vi "HapticSTM_FBL.vi"() -> ()   [LabVIEW 2019]
uses:
  <userlib>/HapticSTM/HapticSTM.lvlib
  SubVIs/GlobalClicksHeight_FBL.vi
  <vilib>/sound2/lvsound2.llb/Sampling Mode.ctl
  <vilib>/sound2/lvsound2.llb/Sound Data Format.ctl
  <vilib>/sound2/lvsound2.llb/Sound Output Write (DBL Single).vi
  <vilib>/sound2/lvsound2.llb/Sound Output Set Volume (Single).vi
panel:
  in  "Surface Location (nm)":dbl
  in  "Z Write?":bool
  in  "Planing?":bool
  in  "Plunge Depth (pm)":dbl=280.0 format="%.1f"
  out "Button":bool
  out "Setpoint (pA)":dbl
  in  "Maximum (pA)":dbl=9000.0
  out "Filtered Current (pA)":dbl format="%.1f"
  out "Current (pA)":dbl format="%.1f"
  out "Oy":dbl
  out "Ox":dbl
  out "W":dbl
  out "H":dbl
  out "Z Write (m)":dbl format="%^.1e"
  out "Z Read (m)":dbl format="%^#.1e"
  out "Vy":dbl format="%.1f"
  out "Vz":dbl format="%.1f"
  out "Vx":dbl format="%.1f"
  out "Fy":dbl format="%.1f"
  out "Fz":dbl format="%.1f"
  out "Fx":dbl format="%.1f"
  out "phi":dbl format="%.1f"
  out "psi":dbl format="%.1f"
  out "theta":dbl format="%.1f"
  out "x":dbl format="%.1f"
  out "y":dbl format="%.1f"
  out "z":dbl format="%0.1f"
  out "Height":dbl format="%^.1e"
  in  "Hardness":dbl=1.0 format="%.1f"
  in  "Mode":u16(ring) items=["Log w/ Exp Z", "Log w/ Lin Z"]
  in  "Reset Clicks":bool
  out "Clicks":i32
  in  "STOP":bool
  in  "START":bool
  out "Seq":i32
  out "SeqString":string
  out "Raw and Scaled Z Positions":cluster{dbl, "Y":dbl}(graph)
  out "Scaled Force and Current":T1(graph)
  in  "Sensitivity":dbl=1.0 format="%.1f"
  in  "Volume":dbl(slide)=50.0 scale=0.0..100.0
  in  "Device ID":u32
  # "Nanonis"
  # "No"
  # "Yes"
  # "Current"
  # "Frame"
  # "Z Controller"
  # "Haptic Pen"
  # "Position"
  # "Force"
  # "Angles"
  # "Velocity"
  # "Surface"
  # "Clicks"
  # "Haptic STM Controller 3000"
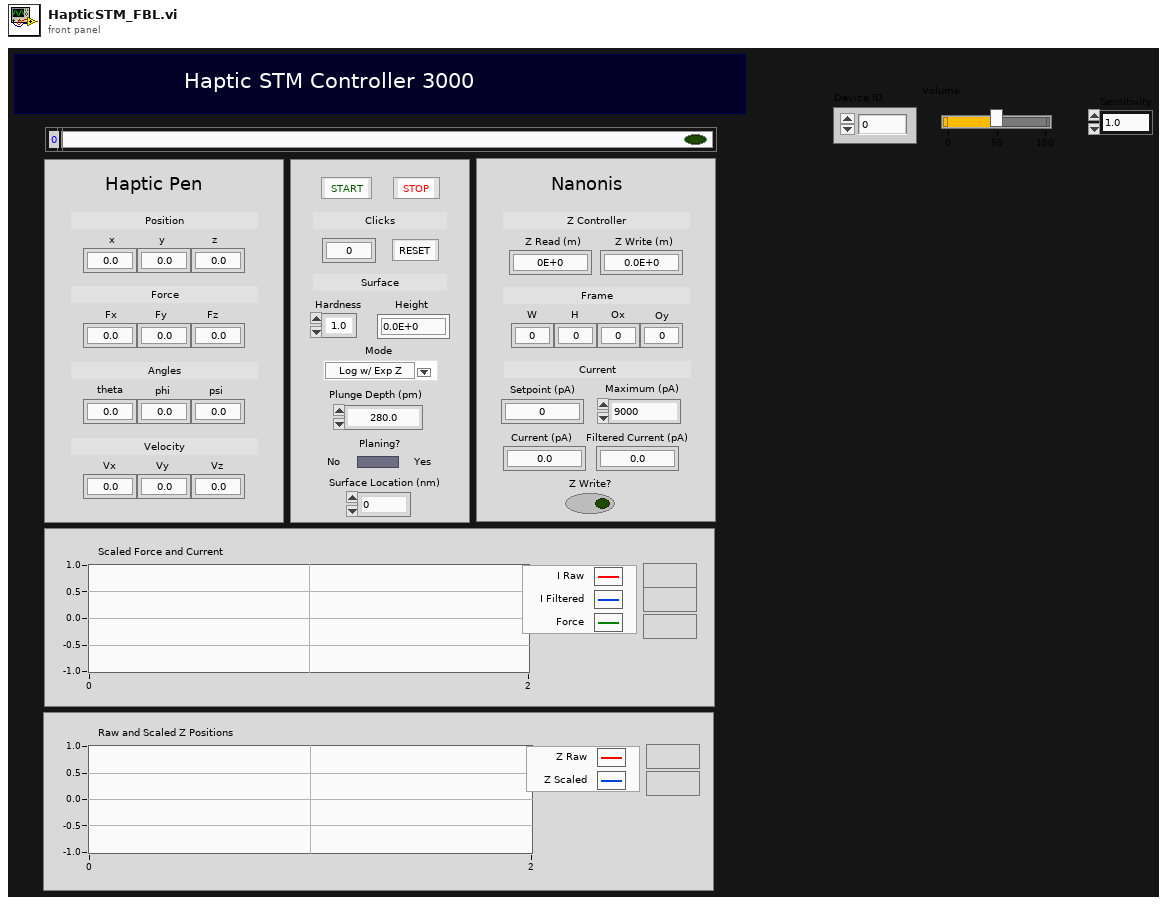
[diagram p1: front panel]
types:
  T1 = cluster{"Current (pA)":sgl, "Filtered Current (pA)":dbl, dbl}
  T2 = typedef "Sound Data Format.ctl" = cluster{"sample rate (S/s)":dbl, "number of channels":i32, "bits per sample":i32}
  T3 = typedef "Sampling Mode.ctl" = i32
  T4 = typedef "Sound Output Task ID.ctl" = u32
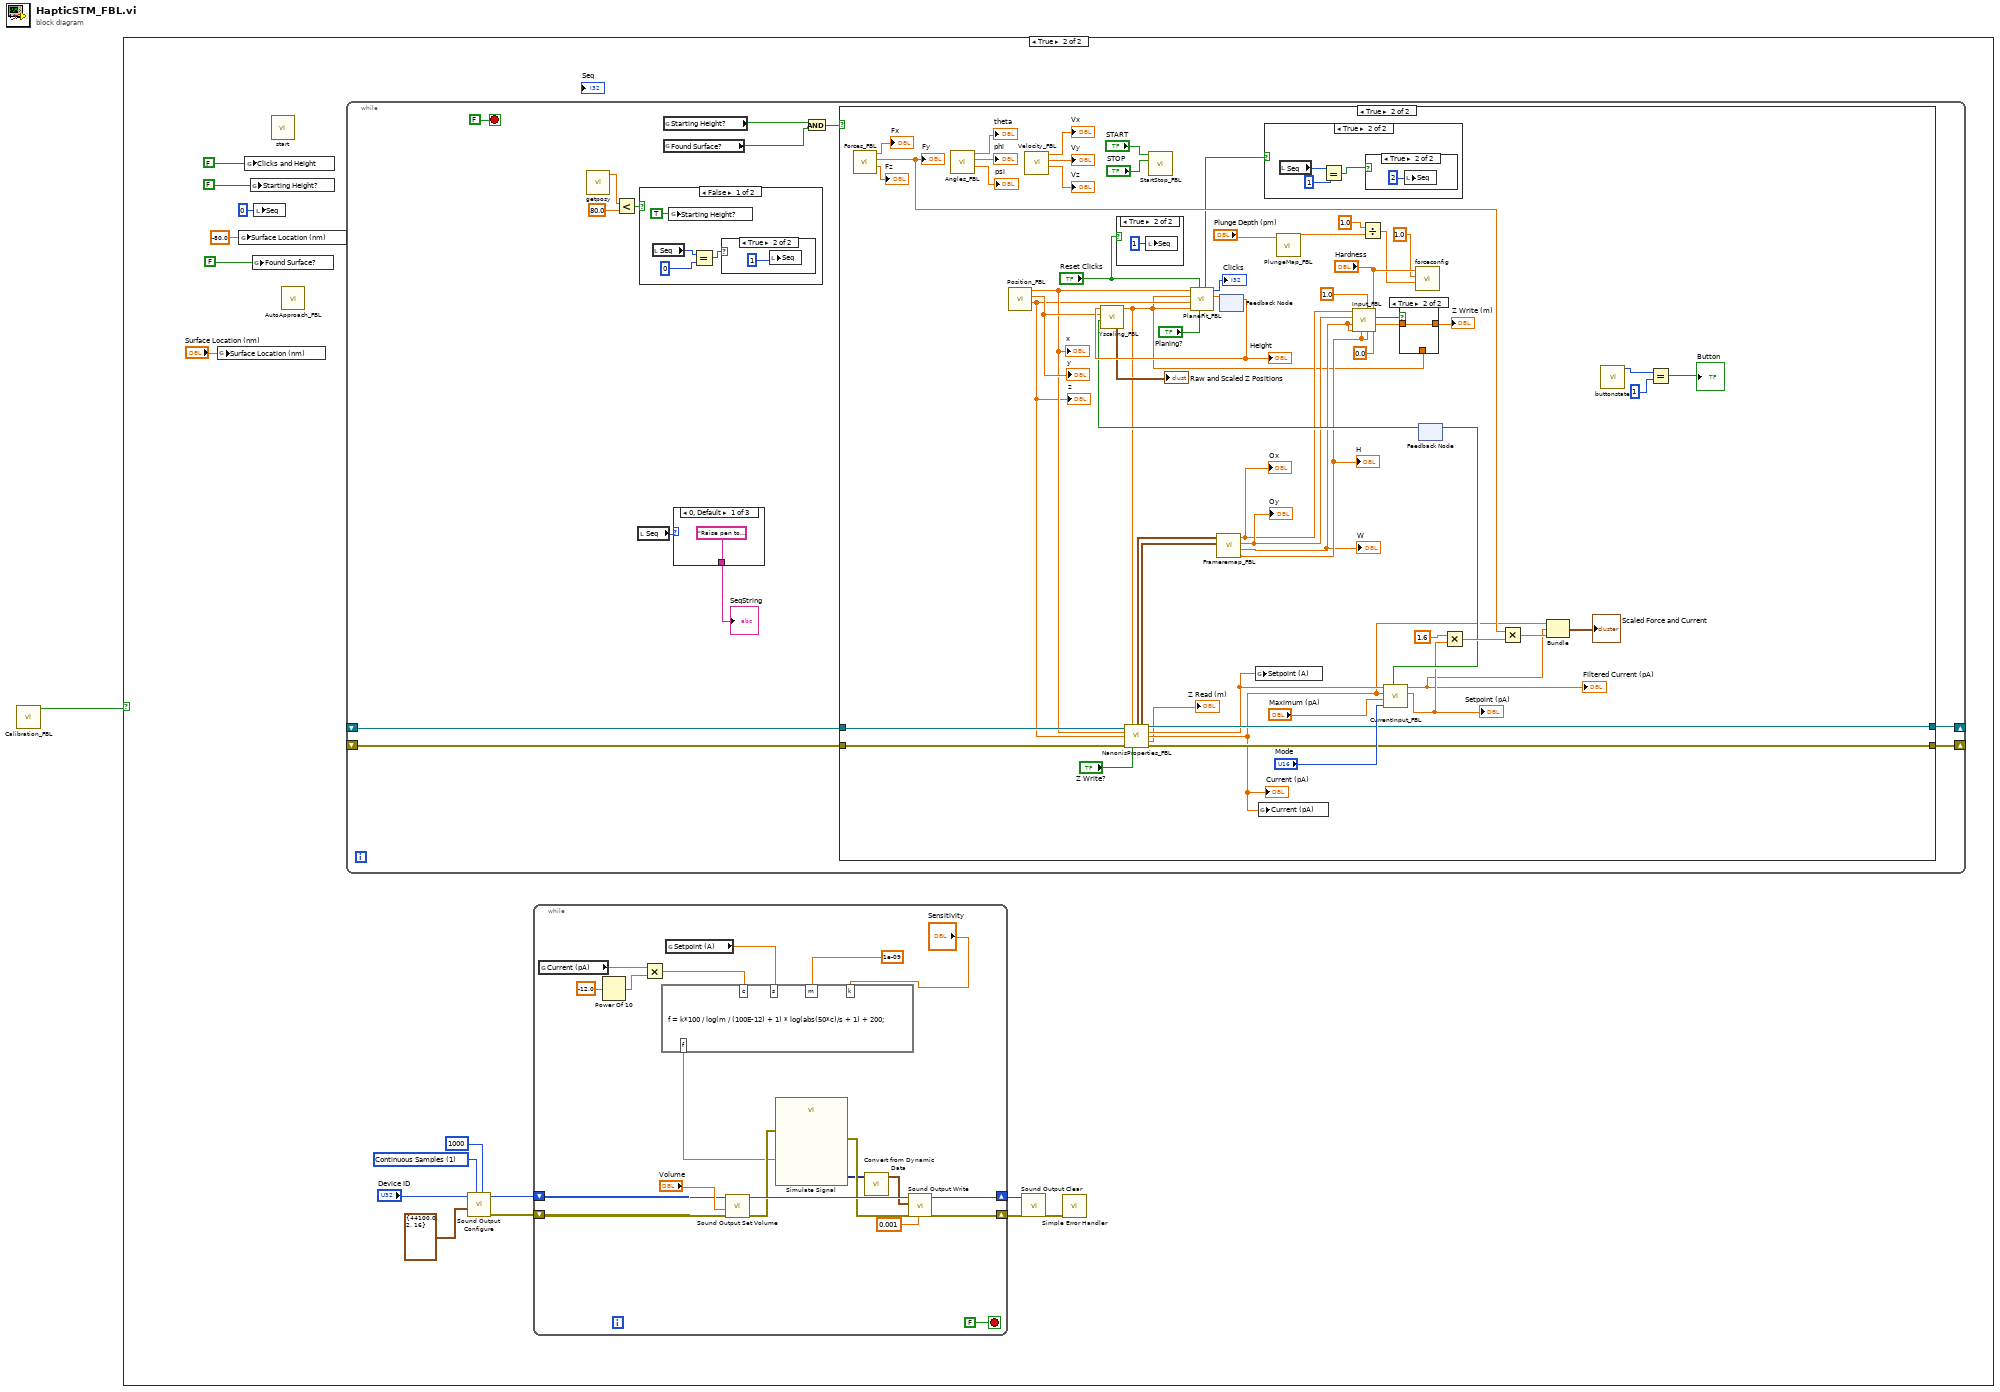
[diagram p0: block diagram]
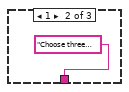
[diagram p3: hidden frame]
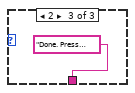
[diagram p4: hidden frame]
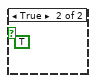
[diagram p6: hidden frame]
diagram:
  n1 = call "Calibration_FBL.vi"() -> ("Calibration Complete?"=w1:bool)  [unwired: 11 in]
  n2 = case shown="True" w1 {
    frame False {
    }
    frame True {
      w10 = T3 1 items=["Finite Samples", "Continuous Samples"] ("sample mode")
      n3 = global write "GlobalClicksHeight_FBL.vi" "Surface Location (nm)"("Surface Location (nm)") -> ()
      n4 = global write "GlobalClicksHeight_FBL.vi" "Surface Location (nm)"(-80.0 ("Surface Location")) -> ()
      n5 = global write "GlobalClicksHeight_FBL.vi" "Clicks and Height"(FALSE ("Clicks and Height")) -> ()
      n6 = global write "GlobalClicksHeight_FBL.vi" "Starting Height?"(FALSE ("Clicks and Height")) -> ()
      n7 = global write "GlobalClicksHeight_FBL.vi" "Found Surface?"(FALSE ("Clicks and Height")) -> ()
      n8 = local write "Seq"(0 ("Seq")) -> ()
      n9 = call <userlib>:"start.vi"() -> ()  [unwired: 11 in, 1 out]
      n10 = call "AutoApproach_FBL.vi"() -> ()  [unwired: 12 in]
      n11 = while {
        shift-right: [w39] -> _
        shift-left: _ -> [w40]
        shift-right: [w38] -> _
        shift-left: _ -> [w37]
        stop <- FALSE stop-if-true
        n12 = call <userlib>:"getposy.vi"() -> ("function return"=w49:dbl)  [unwired: 11 in]
        n13 = Less?(x=w49, y=80.0) -> (x < y?=w47:bool)
        n14 = local read "Seq"() -> (w45:i32)
        n15 = case shown="False" w47 {
          frame False {
            n16 = local read "Seq"() -> (w55:i32)
            n17 = global write "GlobalClicksHeight_FBL.vi" "Starting Height?"(TRUE ("Starting Height?")) -> ()
            n18 = Equal?(x=w55, y=0) -> (x = y?=w53:bool)
            n19 = case shown="True" w53 {
              frame False {
              }
              frame True {
                n20 = local write "Seq"(1 ("Seq")) -> ()
              }
            }
          }
          frame True {
            (unwired) TRUE ("Clicks and Height")
          }
        }
        n21 = global read "GlobalClicksHeight_FBL.vi" "Starting Height?"() -> (w42:bool)
        n22 = global read "GlobalClicksHeight_FBL.vi" "Found Surface?"() -> (w41:bool)
        n23 = case shown="0, Default" w45 {
          tunnel: ["Raise pen to begin." "Choose three points, then raise the arm to plane." "Done. Press 'STOP' to stop at anytime."] -> w44
          frame 0, Default {
          }
          frame 1 {
          }
          frame 2 {
          }
        }
        "SeqString" <- w44
        n24 = And(x=w42, y=w41) -> (x .and. y?=w43:bool)
        n25 = case shown="True" w43 {
          tunnel: w40 -> [_ w72]
          tunnel: [_ w71] -> w39
          tunnel: [_ w70] -> w38
          tunnel: w37 -> [_ w69]
          frame False {
          }
          frame True {
            n26 = call "Forces_FBL.vi"() -> ("Fz"=→"Fz":dbl, "Fy"=w102:dbl, "Fx"=→"Fx":dbl)  [unwired: 9 in]
            "Fy" <- w102
            n27 = call "Angles_FBL.vi"() -> ("psi"=→"psi":dbl, "phi"=→"phi":dbl, "theta"=→"theta":dbl)  [unwired: 9 in]
            n28 = call "Position_FBL.vi"() -> ("Z"=w67:dbl, "Y"=w98:dbl, "X"=w68:dbl)  [unwired: 9 in]
            "x" <- w68
            "y" <- w98
            "z" <- w67
            n29 = call "Velocity_FBL.vi"() -> ("VZ"=→"Vz":dbl, "VY"=→"Vy":dbl, "VX"=→"Vx":dbl)  [unwired: 9 in]
            n30 = case shown="True" "Reset Clicks" {
              frame False {
              }
              frame True {
                n31 = local write "Seq"(1 ("Seq")) -> ()
              }
            }
            n32 = call "StartStop_FBL.vi"("STOP"="STOP", "START"="START") -> ()  [unwired: 10 in]
            n33 = feedback #1() -> (w105:dbl)  [unwired: 1 in]
            "Height" <- w105
            n34 = call "PlungeMap_FBL.vi"("Input (pA)"="Plunge Depth (pm)") -> ("output"=w59:dbl)  [unwired: 10 in]
            n35 = Divide(x=1.0, y=w59) -> (x/y=w83:dbl)
            n36 = call <userlib>:"forceconfig.vi"("c"=w83, "b"=1.0, "a"="Hardness") -> ()  [unwired: 9 in]
            n37 = feedback #2() -> (w104:bool)  [unwired: 1 in]
            n38 = call "Yscaling_FBL.vi"("Current Maxed?"=w104, "Y"=w98, "Plane Height"=w105) -> ("y scaled (m)"=w63:dbl, "Zpos Graph (nm)"=→"Raw and Scaled Z Positions":cluster{dbl, "function return":dbl})  [unwired: 7 in]
            n39 = call "NanonisProperties_FBL.vi"("Application reference"=w69, "Z Write (m)"=w63, "X pen (nm)"=w68, "Z pen (nm)"=w67, "Error in"=w72, "Z Write?"="Z Write?") -> ("Frame Size (m)"=w61:cluster{"Width":sgl, "Height":sgl}, "Frame Origin (m)"=w62:cluster{"Xc":sgl, "Yc":sgl}, "Application ref out"=w70:refnum<vi>, "Setpoint (pA)"=w66:sgl, "Current (pA)"=w65:sgl, "Z Read (m)"=→"Z Read (m)":sgl, "error out"=w71:errorcluster)  [unwired: 3 in]
            "Current (pA)" <- w65
            n40 = call "PlaneFit_FBL.vi"("Planing y/n?"="Planing?", "Reset Clicks"="Reset Clicks", "Y PEN"=w63, "Z"=w67, "Nano Z"=w63, "X"=w68) -> ("Plane Height (m)"=w106:dbl, "Clicks"=→"Clicks":i32, "Planing Done?"=w91:bool)  [unwired: 3 in]
            n41 = call "Frameremap_FBL.vi"("Frame Origin (m)"=w62, "Frame Size (m)"=w61) -> ("FH"=w82:dbl, "FW"=w81:dbl, "Z Origin"=w80:dbl, "X Origin"=w79:dbl)  [unwired: 6 in]
            "H" <- w82
            "W" <- w81
            "Ox" <- w79
            "Oy" <- w80
            n42 = feedback-in #1(w106) -> ()
            n43 = global write "GlobalClicksHeight_FBL.vi" "Setpoint (A)"(w66) -> ()
            n44 = global write "GlobalClicksHeight_FBL.vi" "Current (pA)"(w65) -> ()
            n45 = case shown="True" w91 {
              frame False {
              }
              frame True {
                n46 = local read "Seq"() -> (w123:i32)
                n47 = Equal?(x=w123, y=1) -> (x = y?=w121:bool)
                n48 = case shown="True" w121 {
                  frame False {
                  }
                  frame True {
                    n49 = local write "Seq"(2 ("Seq")) -> ()
                  }
                }
              }
            }
            n50 = call "Input_FBL.vi"("Current * 10^input"=0.0, "Sensitivity"="Hardness", "Scopez"=w82, "Drag"=1.0, "FH"=w82, "FW"=w81, "Scopex"=w81, "Z origin"=w80, "X origin"=w79) -> ("Scaled Current"=w85:dbl, "feedback"=w87:bool)  [unwired: 1 in]
            n51 = call "CurrentInput_FBL.vi"("Mode"="Mode", "Maximum (pA)"="Maximum (pA)", "Current (pA)"=w65, "Setpoint (A)"=w66) -> ("Setpoint (pA)"=w74:dbl, "Filtered Current (pA)"=w73:dbl, "Current Maxed?"=w75:bool)  [unwired: 5 in]
            "Filtered Current (pA)" <- w73
            "Setpoint (pA)" <- w74
            n52 = case shown="True" w87 {
              tunnel: [w118 w119] -> w86
              tunnel: w85 -> [_ w119]
              tunnel: w63 -> [w118 _]
              frame False {
              }
              frame True {
              }
            }
            "Z Write (m)" <- w86
            n53 = feedback-in #2(w75) -> ()
            n54 = Multiply(x=1.6 ("y"), y=w74) -> (x*y=w99:dbl)
            n55 = Multiply(x=w102, y=w99) -> (x*y=w101:dbl)
            n56 = Bundle("Current (pA)"=w65, "Filtered Current (pA)"=w73, w101) -> (→"Scaled Force and Current":T1)  [unwired: 1 in]
            n57 = call <userlib>:"buttonstate.vi"() -> ("function return"=w97:i32)  [unwired: 11 in]
            n58 = Equal?(x=w97, y=1) -> (x = y?=→"Button":bool)
          }
        }
      }
      n59 = call <vilib>:"Sound Output Configure.vi"("number of samples/ch"=1000 ("Number of Samples/ch"), "sample mode"=w10, "sound format"=T2 {"sample rate (S/s)"=44100.0, "number of channels"=2, "bits per sample"=16} ("Sound Format"), "device ID"="Device ID") -> ("error out"=w6:errorcluster, "task ID"=w7:T4)  [unwired: 6 in]
      n60 = while {
        shift-right: [w28] -> w5
        shift-left: w7 -> [w30]
        shift-right: [w27] -> w4
        shift-left: w6 -> [w29]
        stop <- FALSE stop-if-true
        n61 = global read "GlobalClicksHeight_FBL.vi" "Current (pA)"() -> (w19:dbl)
        n62 = Power Of 10(x=-12.0) -> (10^x=w21:dbl)
        n63 = Multiply(x=w19, y=w21) -> (x*y=w18:dbl)
        n64 = global read "GlobalClicksHeight_FBL.vi" "Setpoint (A)"() -> (w23:dbl)
        n65 = formula code="f = k*100 / log(m / (100E-12) + 1) * log(abs(50*c)/s + 1) + 200;"("c"=w18, "m"=1e-09 ("input variable"), "s"=w23, "k"="Sensitivity") -> ("f"=w22:dbl)
        n66 = call-poly <vilib>:"Sound Output Set Volume.vi"("error in (no error)"=w29, "volume"="Volume", "task ID"=w30) -> ("error out"=w33:errorcluster, "task ID out"=w36:T4)  [unwired: 7 in]
        n67 = call "Simulate Signal"("Frequency"=w22, "error in (no error)"=w33) -> ("Sine"=w31:dynamicdata, "error out"=w32:errorcluster)  [unwired: 12 in]
        n68 = call "Convert from Dynamic Data"("Dynamic Data Type"=w31) -> ("Waveform"=w34:waveform(dbl))  [unwired: 3 in]
        n69 = call-poly <vilib>:"Sound Output Write.vi"("timeout (sec)"=0.001, "error in (no error)"=w32, "data"=w34, "task ID"=w36) -> ("error out"=w27:errorcluster, "task ID out"=w28:T4)  [unwired: 6 in]
      }
      n70 = call <vilib>:"Sound Output Clear.vi"("error in (no error)"=w4, "task ID"=w5) -> ("error out"=w9:errorcluster)  [unwired: 9 in]
      n71 = call <vilib>:"Simple Error Handler.vi"("error in (no error)"=w9) -> ()  [unwired: 4 in, 5 out]
    }
  }
